vi "保存电子表格文件.vi"() -> ()   [LabVIEW 2010]
uses:
  <vilib>/Utility/file.llb/Write To Spreadsheet File (DBL).vi
panel:
  in  "路径":path
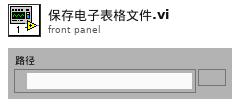
[diagram p1: front panel]
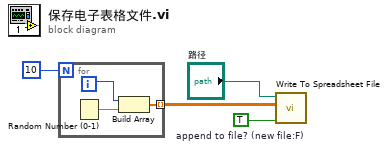
[diagram p0: block diagram]
diagram:
  w4 = TRUE  # append to file? (new file:F)
  n1 = for {
    N: 10 -> [_]
    tunnel: [w7] -> w3 mode=indexing
    i -> [w6]
    n2 = Random Number (0-1)() -> (number: 0 to 1=w5:dbl)
    n3 = Build Array(w6, w5) -> (w7:dbl[])
  }
  n4 = call-poly <vilib>:"Write To Spreadsheet File.vi"("append to file? (new file:F)"=w4, "2D data"=w3, "file path (dialog if empty)"="路径") -> ()  [unwired: 5 in, 1 out]
